vi "Left Guitar Green.vi"(0 "ROI Descriptor (Line Profile 1)":T1={"Global Rectangle"=[91, 296, 132, 392], "Contours"=[{"ID"=enum."External", "Type"=2, "Coordinates"=[131, 296, 91, 391]}]} {"Contours"."Type" items=["No Selection", "Point", "Line", "Rectangle", "Oval", "Polygon", "Freehand Region", "Annulus", "Unused2", "Unused3", "Broken Line", "Freehand Line", "Rotated Rectangle"]}, 1 "Color Mode (Line Profile 1)":u16(ring)=3 items=["RGB", "HSL", "HSV", "HSI"], 2 "File Path":path, 7 "error in":errorcluster) -> (20 "Line Profile (Line Profile 1)":u8[][](array[numeric]), 27 "error out":errorcluster)   [LabVIEW 2009]
panel:
  out "Image Out":T2(plugin-control)
  out "Line Profile Graph":u8[][](graph) caption="Line Profile"
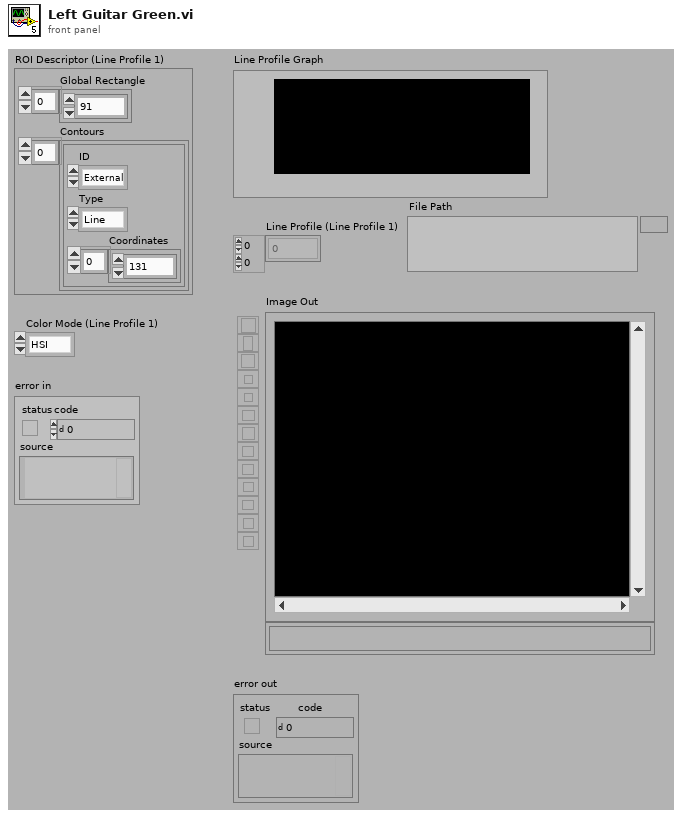
[diagram p1: front panel]
types:
  T1 = cluster{"Global Rectangle":i32[], "Contours":cluster{"ID":enum32{"External", "Internal"}, "Type":u32, "Coordinates":i32[]}[]}
  T2 = typedef "IMAQ Image.ctl" = refnum<image>
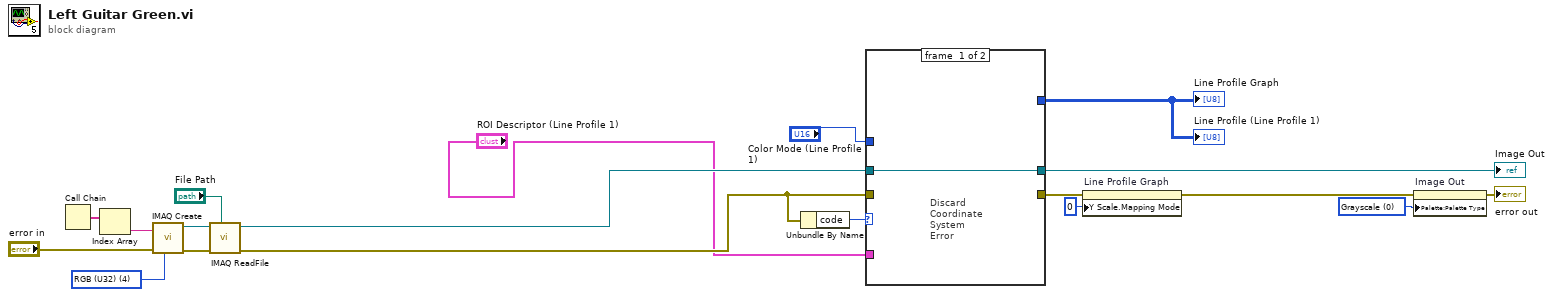
[diagram p0: block diagram]
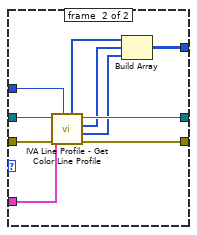
[diagram p2: hidden frame]
diagram:
  w3 = u32 0 items=["Grayscale", "Binary", "Gradient", "Rainbow", "Temperature", "User Defined"] ("Palette")
  w16 = u32 4 items=["Grayscale (U8)", "Grayscale (I16)", "Grayscale (SGL)", "Complex (CSG)", "RGB (U32)", "HSL (U32)", "RGB (U64)"] ("Image Type")
  n1 = Call Chain() -> (call chain=w14:string[])
  n2 = Index Array(array=w14) -> (element=w13:string)  [unwired: 1 in]
  n3 = call "IMAQ Create"("Image Name"=w13, "Image Type"=w16, "error in (no error)"="error in") -> ("New Image"=w18:T2, "error out"=w17:errorcluster)  [unwired: 1 in, 1 out]
  n4 = call "IMAQ ReadFile"("File Path"="File Path", "error in (no error)"=w17, "Image"=w18) -> ("error out"=w19:errorcluster, "Image Out"=w8:T2)  [unwired: 2 in, 5 out]
  n5 = Unbundle By Name(w19) -> ("code"=w5:i32)
  n6 = case shown="Default" w5 {
    tunnel: w19 -> [_ w30]
    tunnel: [_ w29] -> w11
    tunnel: "Color Mode (Line Profile 1)" -> [_ w28]
    tunnel: [w20 w27] -> w4
    tunnel: w8 -> [w20 w26]
    tunnel: [_ w22] -> w7
    tunnel: "ROI Descriptor (Line Profile 1)" -> [_ w21]
    frame #0 {
      # "Discard\nCoordinate\nSystem\nError"
    }
    frame #1 {
      n7 = call <vilib>:"IVA Line Profile - Get Color Line Profile.vi"("Color Mode"=w28, "error in (no error)"=w30, "ROI Descriptor"=w21, "Image In"=w26) -> ("error out"=w29:errorcluster, "Blue or Luma Pixels"=w23:u8[], "Green or Sat Pixels"=w24:u8[], "Image Out"=w27:T2, "Red or Hue Pixels"=w25:u8[])  [unwired: 3 out]
      n8 = Build Array(w25, w24, w23) -> (w22:u8[][])
    }
  }
  "Line Profile Graph" <- w7
  "Line Profile (Line Profile 1)" <- w7
  "Image Out" <- w4
  n9 = property on="Line Profile Graph"(error in=w11, "Y Scale.Mapping Mode"=u8 0) -> (error out=w10:errorcluster)  [unwired: 1 in, 1 out]
  n10 = property on="Image Out" class="ImageControl"(error in=w10, "Palette:Palette Type"=w3) -> (error out=→"error out":errorcluster)  [unwired: 1 in, 1 out]
